vi "deleteLastLine.vi"(6 "TypeControl":bool, 8 "error in (no error)":errorcluster, 11 "XuLyDataDisplay in":refnum<class "XuLyDataDisplay.lvclass">) -> (0 "error out":errorcluster, 3 "XuLyDataDisplay out":refnum<class "XuLyDataDisplay.lvclass">)   [LabVIEW 2017, in "LibraryGcode.lvlib" / "XuLyDataDisplay.lvclass"]
uses:
  XuLyDataDisplay.lvclass
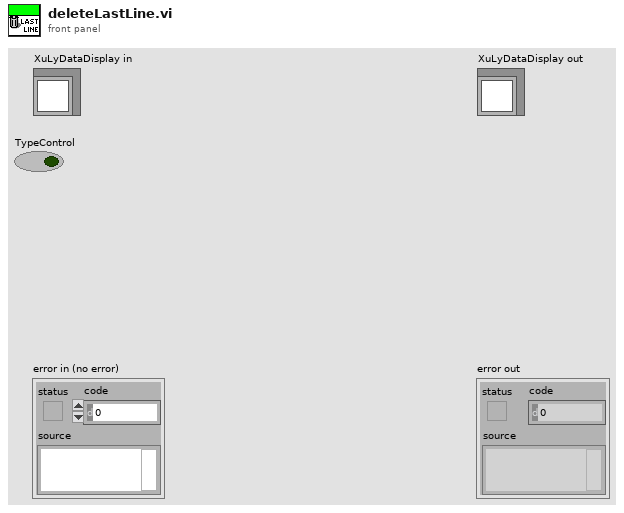
[diagram p1: front panel]
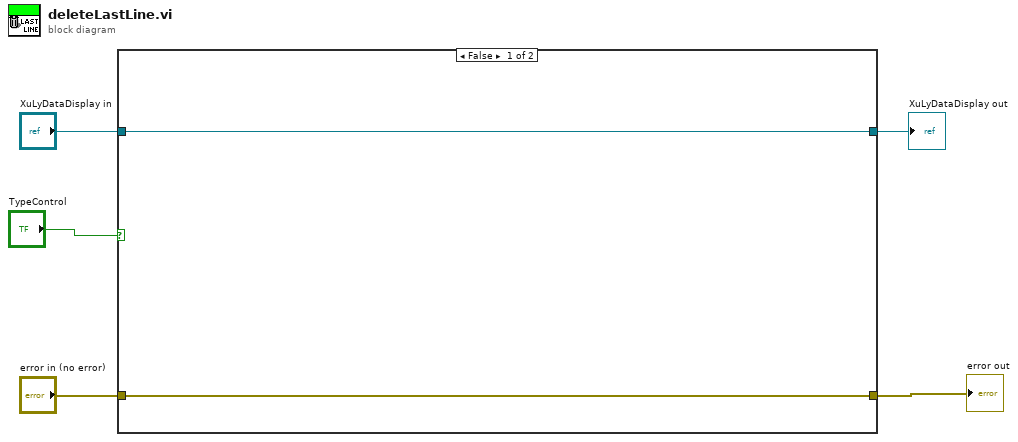
[diagram p0: block diagram]
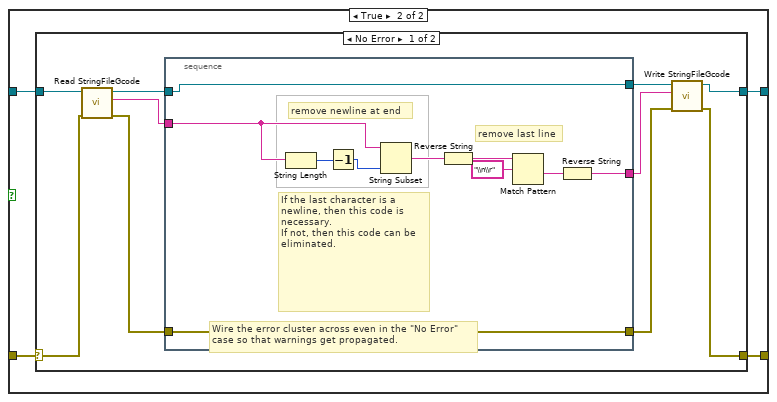
[diagram p2: hidden frame]
diagram:
  n1 = case shown="False" "TypeControl" {
    tunnel: "error in (no error)" -> [w6 w11]
    tunnel: [w6 w10] -> w4
    tunnel: "XuLyDataDisplay in" -> [w7 w9]
    tunnel: [w7 w8] -> w2
    frame False {
    }
    frame True {
      n2 = case shown="No Error" w11 {
        selector: w11 -> [w20 w33]
        tunnel: [w14 w33] -> w10
        tunnel: [w16 w32] -> w8
        tunnel: w9 -> [w21 w32]
        frame No Error {
          # "Wire the error cluster across even in the \"No Error\"\ncase so that warnings get propagated."
          n3 = call-dynamic "Read StringFileGcode.vi"("error in (no error)"=w20, "ParameterConf in"=w21) -> ("error out"=w17:errorcluster, "StringFileGcode"=w18:string, "ParameterConf out"=w19:refnum<class "XuLyDataDisplay.lvclass">)  [unwired: 7 in]
          n4 = stacked-sequence {
            tunnel: w18 -> [w26]
            tunnel: [w25] -> w12
            tunnel: w19 -> [w22]
            tunnel: [w23] -> w13
            tunnel: w17 -> [w23]
            tunnel: [w22] -> w15
            frame #0 {
              # "remove last line"
              # "remove newline at end"
              # "If the last character is a newline, then this code is necessary.\nIf not, then this code can be eliminated."
              n5 = String Length(string=w26) -> (length=w29:i32)
              n6 = Decrement(x=w29) -> (x-1=w31:i32)
              n7 = String Subset(string=w26, length (rest)=w31) -> (substring=w30:string)  [unwired: 1 in]
              n8 = Reverse String(1:w30) -> (0:w27:string)
              n9 = Match Pattern(string=w27, regular expression="\\n\\r") -> (after substring=w28:string)  [unwired: 1 in, 3 out]
              n10 = Reverse String(1:w28) -> (0:w25:string)
            }
          }
          n11 = call-dynamic "Write StringFileGcode.vi"("error in (no error)"=w13, "StringFileGcode"=w12, "ParameterConf in"=w15) -> ("error out"=w14:errorcluster, "ParameterConf out"=w16:refnum<class "XuLyDataDisplay.lvclass">)  [unwired: 7 in]
        }
        frame Error {
        }
      }
    }
  }
  "error out" <- w4
  "XuLyDataDisplay out" <- w2
